vi "Parse messages.vi"(8 "error in (no error)":errorcluster, 11 "JSON (UTF-8) String":string) -> (0 "error out":errorcluster, 2 "Telegram State":T1, 3 "Variant":variant)   [LabVIEW 2015, in "JSON Library.lvlib"]
doc: "Created IvanLis by LabVIEW Portal\nProfile: http://labviewportal.org/memberlist.php?mode=viewprofile&u=987\neMail: IvanLisanov@gMail.com\nTelegram: https://t.me/IvanLis"
uses:
  JSON Library.lvlib
  Telegram Library/TypeDef/Telegram State.ctl
  TypeDef/Message Text.ctl
  Telegram Library/Telegram Library.lvlib
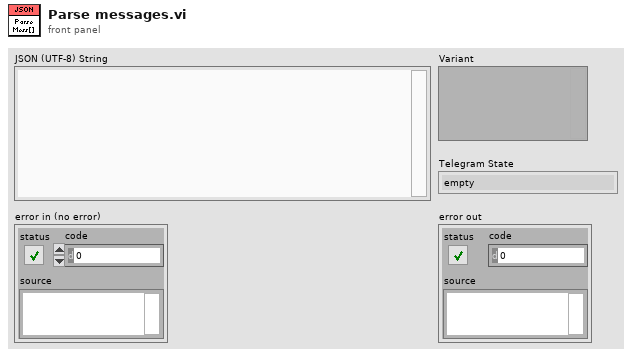
[diagram p1: front panel]
types:
  T1 = typedef "Telegram Library.lvlib/Telegram State.ctl" = enum16{"empty", "ok", "authorizationStateClosed", "authorizationStateWaitTdlibParameters", "authorizationStateWaitEncryptionKey", "authorizationStateWaitPhoneNumber", "authorizationStateWaitCode", "connectionStateWaitingForNetwork", "connectionStateConnectingToProxy", "connectionStateUpdating", "connectionStateConnecting", "connectionStateReady", "updateUser_user", "updateNewChat_chat", "updateNewMessage_Text", "updateChatLastMessage_Text", "updateDeleteMessages", "updateChatPosition", "ChatHistoryMessages_Text"}
  T2 = typedef "JSON Library.lvlib/Message Text.ctl" = cluster{"@type":string, "id":i64, "sender_id":cluster{"@type":string, "user_id":i64}, "chat_id":i64, "date":i64, "content":cluster{"@type":string, "text":cluster{"@type":string, "text":string}}}
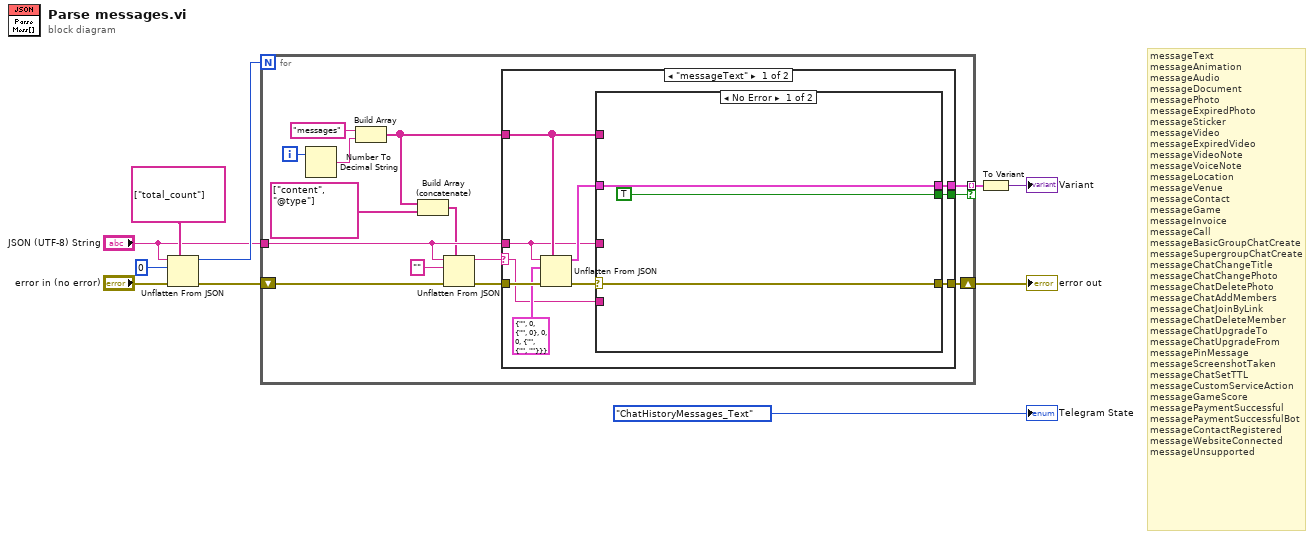
[diagram p0: block diagram]
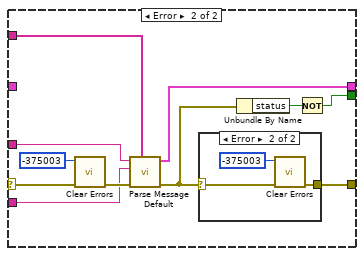
[diagram p2: hidden frame]
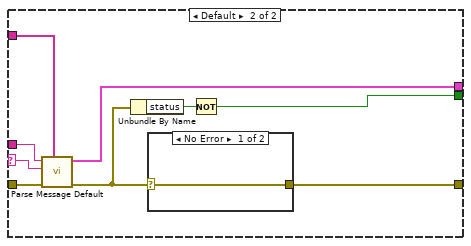
[diagram p4: hidden frame]
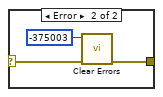
[diagram p5: hidden frame]
diagram:
  # "messageText\nmessageAnimation\nmessageAudio\nmessageDocument\nmessagePhoto\nmessageExpiredPhoto\nmessageSticker\nmessageVideo\nmessageExpiredVideo\nmessageVideoNote\nmessageVoiceNote\nmessageLocation\nmessageVenue\nmessageContact\nmessageGame\nmessageInvoice\nmessageCall\nmessageBasicGroupChatCreate\nmessageSupergroupChatCreate\nmessageChatChangeTitle\nmessageChatChangePhoto\nmessageChatDeletePhoto\nmessageChatAddMembers\nmessageChatJoinByLink\nmessageChatDeleteMember\nmessageChatUpgradeTo\nmessageChatUpgradeFrom\nmessagePinMessage\nmessageScreenshotTaken\nmessageChatSetTTL\nmessageCustomServiceAction\nmessageGameScore\nmessagePaymentSuccessful\nmessagePaymentSuccessfulBot\nmessageContactRegistered\nmessageWebsiteConnected\nmessageUnsupported"
  n1 = Unflatten From JSON(path=string[] ["total_count"], JSON string="JSON (UTF-8) String", type and defaults=0, error in (no error)="error in (no error)") -> (value=w9:i32, error out=w5:errorcluster)  [unwired: 3 in]
  n2 = for {
    N: w9 -> [_]
    tunnel: "JSON (UTF-8) String" -> [w17]
    tunnel: [w23] -> w6 mode=indexing if=w11
    shift-right: [w24] -> w1
    shift-left: w5 -> [w18]
    i -> [w22]
    n3 = Number To Decimal String(number=w22) -> (decimal integer string=w20:string)  [unwired: 1 in]
    n4 = Build Array("messages", w20) -> (w12:string[])
    n5 = Build Array (concatenate)(w12, string[] ["content", "@type"] ("path")) -> (w15:string[])
    n6 = Unflatten From JSON(path=w15, JSON string=w17, type and defaults="", error in (no error)=w18) -> (value=w13:string, error out=w16:errorcluster)  [unwired: 3 in]
    n7 = case shown="\"messageText\"" w13 {
      selector: w13 -> [w26 w59]
      tunnel: w16 -> [w34 w60]
      tunnel: [w31 w53] -> w24
      tunnel: [w29 w56] -> w23
      tunnel: w17 -> [w25 w58]
      tunnel: w12 -> [w27 w57]
      tunnel: [w32 w61] -> w11
      frame "messageText" {
        n8 = Unflatten From JSON(path=w27, JSON string=w25, type and defaults=T2 {"@type"="", "id"=0, "sender_id"={"@type"="", "user_id"=0}, "chat_id"=0, "date"=0, "content"={"@type"="", "text"={"@type"="", "text"=""}}} ("New Message Text"), error in (no error)=w34) -> (value=w28:T2, error out=w30:errorcluster)  [unwired: 3 in]
        n9 = case shown="No Error" w30 {
          selector: w30 -> [w35 w43]
          tunnel: [TRUE w47] -> w32
          tunnel: [w35 w46] -> w31
          tunnel: w28 -> [w37 _]
          tunnel: [w37 w38] -> w29
          tunnel: w27 -> [_ w42]
          tunnel: w26 -> [_ w41]
          tunnel: w25 -> [_ w40]
          frame No Error {
          }
          frame Error {
            n10 = call <vilib>:"Clear Errors.vi"("error in (no error)"=w43, "specific error code to clear (0: all)"=-375003) -> ("error out"=w44:errorcluster)  [unwired: 4 in, 1 out]
            n11 = call "Parse Message Default.vi"("path"=w42, "error in (no error)"=w44, "content.@type"=w41, "JSON (UTF-8) String"=w40) -> ("error out"=w39:errorcluster, "New Message Text"=w38:T2)  [unwired: 6 in]
            n12 = case shown="Error" w39 {
              selector: w39 -> [w49 w52]
              tunnel: [w49 w51] -> w46
              frame No Error {
              }
              frame Error {
                n13 = call <vilib>:"Clear Errors.vi"("error in (no error)"=w52, "specific error code to clear (0: all)"=-375003) -> ("error out"=w51:errorcluster)  [unwired: 4 in, 1 out]
              }
            }
            n14 = Unbundle By Name(w39) -> ("status"=w48:bool)
            n15 = Not(x=w48) -> (.not. x?=w47:bool)
          }
        }
      }
      frame Default {
        n16 = call "Parse Message Default.vi"("path"=w57, "error in (no error)"=w60, "content.@type"=w59, "JSON (UTF-8) String"=w58) -> ("error out"=w54:errorcluster, "New Message Text"=w56:T2)  [unwired: 6 in]
        n17 = Unbundle By Name(w54) -> ("status"=w55:bool)
        n18 = case shown="No Error" w54 {
          selector: w54 -> [w62 w64]
          tunnel: [w62 w63] -> w53
          frame No Error {
          }
          frame Error {
            n19 = call <vilib>:"Clear Errors.vi"("error in (no error)"=w64, "specific error code to clear (0: all)"=-375003) -> ("error out"=w63:errorcluster)  [unwired: 4 in, 1 out]
          }
        }
        n20 = Not(x=w55) -> (.not. x?=w61:bool)
      }
    }
  }
  "error out" <- w1
  n21 = To Variant(anything=w6) -> (Variant=→"Variant":variant)
  "Telegram State" <- Telegram_State."ChatHistoryMessages_Text" ("Telegram State")
